vi "niRFSysCalReader Fetch Cal Tone Power.vi"(8 "error in":errorcluster, 9 "Level (dBm)":dbl, 10 "Frequency (Hz)":dbl, 11 "niRFSysCalReader Handle":T1) -> (0 "error out":errorcluster, 2 "CalTone Power (dBm)":dbl, 3 "niRFSysCalReader Handle out":T1)   [LabVIEW 2017, in "niRFSysCalReader.lvlib"]
doc: "Returns the cal tone power used when calibrating the receiver."
uses:
  niRFSysCalReader.lvlib
  INCLUDES/niRFSysCalReader Handle.ctl
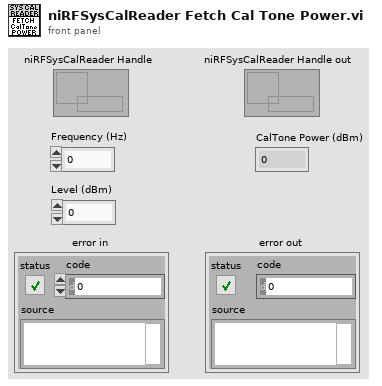
[diagram p1: front panel]
types:
  T1 = typedef "niRFSysCalReader.lvlib/niRFSysCalReader Handle.ctl" = refnum<data-value>
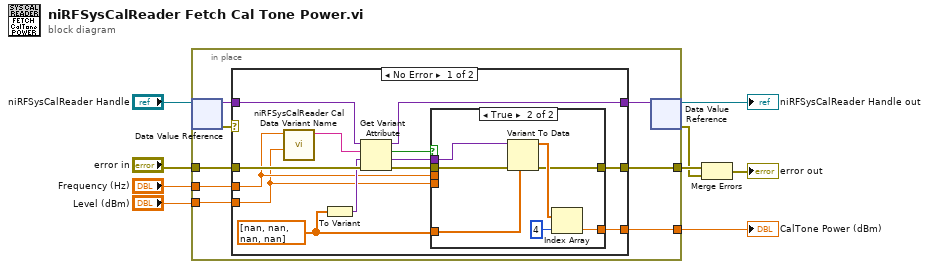
[diagram p0: block diagram]
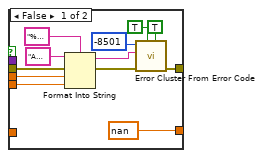
[diagram p2: hidden frame]
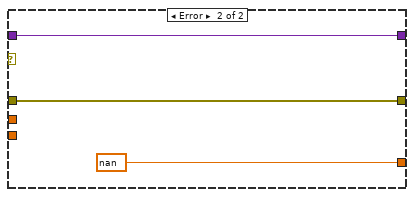
[diagram p3: hidden frame]
diagram:
  n1 = in-place {
    in-place-border: "error in" -> [w16]
    in-place-border: [w13] -> w3
    in-place-border: "Frequency (Hz)" -> [w12]
    in-place-border: "Level (dBm)" -> [w11]
    in-place-border: [w10] -> w5
    n2 = in-place-dvr #1("niRFSysCalReader Handle") -> (w15:variant, w17:errorcluster)
    n3 = case shown="No Error" w17 {
      tunnel: w16 -> [w30 w51]
      tunnel: w15 -> [w28 w52]
      tunnel: [w24 w52] -> w14
      tunnel: [w22 w51] -> w13
      tunnel: w12 -> [w19 _]
      tunnel: w11 -> [w18 _]
      tunnel: [w21 nan] -> w10
      frame No Error {
        w23 = dbl[] [nan, nan, nan, nan]
        n4 = call "niRFSysCalReader Cal Data Variant Name.vi"("Power (dBm)"=w18, "Frequency (Hz)"=w19) -> ("Calibration Data Name"=w29:string)  [unwired: 9 in]
        n5 = To Variant(anything=w23) -> (Variant=w27:variant)
        n6 = Get Variant Attribute(Variant=w28, name=w29, default value (empty Variant)=w27, error in=w30) -> (duplicate Variant=w24:variant, found=w25:bool, value=w20:variant, error out=w26:errorcluster)
        n7 = case shown="True" w25 {
          tunnel: w26 -> [w36 w49]
          tunnel: w23 -> [_ w48]
          tunnel: [w41 w46] -> w22
          tunnel: [nan w45] -> w21
          tunnel: w20 -> [_ w43]
          tunnel: w18 -> [w37 _]
          tunnel: w19 -> [w38 _]
          frame False {
            n8 = Format Into String(format string="%#p Hz, %#f dBm", initial string="A Cal Tone Power value  was not found in the system calibration file at " ("error message (\"\")"), error in=w36, w38, w37) -> (resulting string=w32:string, error out=w35:errorcluster)
            n9 = call <vilib>:"Error Cluster From Error Code.vi"("is warning? (False)"=TRUE, "show call chain? (False)"=TRUE, "error in (no error)"=w35, "error message (\"\")"=w32, "error code (0)"=-8501) -> ("error out"=w41:errorcluster)  [unwired: 4 in]
          }
          frame True {
            n10 = Variant To Data(error in=w49, type=w48, Variant=w43) -> (data=w47:dbl[], error out=w46:errorcluster)
            n11 = Index Array(array=w47, index=4) -> (element=w45:dbl)
          }
        }
      }
      frame Error {
      }
    }
    n12 = in-place-dvr #1(w14) -> (→"niRFSysCalReader Handle out":T1, w1:errorcluster)
  }
  "CalTone Power (dBm)" <- w5
  n13 = Merge Errors(w3, w1) -> (→"error out":errorcluster)
